vi "Start-Stop Remote Ping.vi"(8 "Error In":errorcluster, 10 "Start Remote Ping":bool, 11 "Test LNA in":refnum<class "TestLNA.lvclass">) -> (0 "Error Out":errorcluster, 3 "Test LNA out":refnum<class "TestLNA.lvclass">)   [LabVIEW 2014, in "TestLNA.lvlib" / "TestLNA.lvclass"]
doc: "Start or stop remote ping using iime delayed message."
uses:
  TestLNA.lvclass
  TestLNA.lvclass/TestLNA.ctl
  <vilib>/ActorFramework/Time-Delayed Send Message/Time-Delay Override Options.ctl
  Test LNA Messages/Remote Message Msg/Remote Message Msg.lvclass
  CSPP_Core/Actors/CS++BaseActor/CS++BaseActor.lvclass/CS++BaseActor.ctl
  <vilib>/ActorFramework/Actor/Actor.lvclass/Actor.ctl
  <vilib>/ActorFramework/Message Enqueuer/Message Enqueuer.lvclass/Message Enqueuer.ctl
  <vilib>/ActorFramework/Message Enqueuer/Init from Existing Queue.vi
  <vilib>/ActorFramework/Message Enqueuer/Message Enqueuer.lvclass
  <vilib>/ActorFramework/Actor/Actor.lvclass
  CSPP_Core/Actors/CS++BaseActor/CS++BaseActor.lvclass
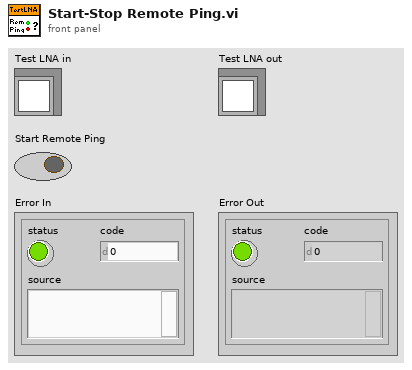
[diagram p1: front panel]
types:
  T1 = typedef "Time-Delay Override Options.ctl" = enum16{"Send next copy now", "Skip next scheduled copy", "Send next copy now and stop all further copies", "Stop all further copies"}
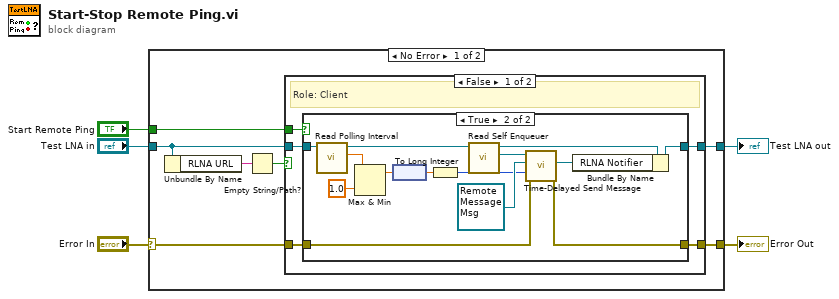
[diagram p0: block diagram]
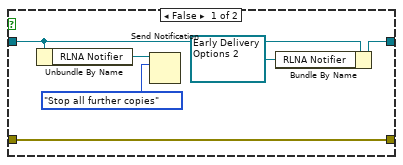
[diagram p2: hidden frame]
diagram:
  n1 = case shown="No Error" "Error In" {
    selector: "Error In" -> [w12 w40]
    tunnel: [w11 w40] -> w4
    tunnel: [w10 w39] -> w2
    tunnel: "Test LNA in" -> [w8 w39]
    tunnel: "Start Remote Ping" -> [w9 _]
    frame No Error {
      n2 = Unbundle By Name(w8) -> ("RLNA URL"=w7:string)
      n3 = Empty String/Path?(string/path=w7) -> (empty?=w6:bool)
      n4 = case shown="False" w6 {
        tunnel: w12 -> [w17 w37]
        tunnel: [w16 w37] -> w11
        tunnel: [w15 w38] -> w10
        tunnel: w9 -> [w14 _]
        tunnel: w8 -> [w13 w38]
        frame False {
          # "Role: Client"
          n5 = case shown="True" w14 {
            tunnel: w17 -> [w18 w34]
            tunnel: [w18 w33] -> w16
            tunnel: w13 -> [w22 w30]
            tunnel: [w21 w32] -> w15
            frame False {
              w20 = refnum<notifier> refnum items=["Send next copy now", "Skip next scheduled copy", "Send next copy now and stop all further copies", "Stop all further copies"] ("RAPing Notifier")
              n6 = Unbundle By Name(w22) -> ("RLNA Notifier"=w23:refnum<notifier>)
              n7 = Send Notification(notification=Time-Delay_Override_Options."Stop all further copies", notifier=w23) -> ()  [unwired: 1 in, 2 out]
              n8 = Bundle By Name(cluster=w22, "RLNA Notifier"=w20) -> (w21:refnum<class "TestLNA.lvclass">)
            }
            frame True {
              n9 = call "Read Polling Interval.vi"("CS++BaseActor in"=w30) -> ("Polling Interval"=w28:dbl[unit], "CS++BaseActor out"=w29:refnum<class "TestLNA.lvclass">)  [unwired: 8 in, 1 out]
              n10 = Max & Min(x=w28, y=dbl[unit] 1.0) -> (max(x,y)=w26:dbl[unit])  [unwired: 1 out]
              n11 = node(w26) -> (w25:dbl)
              n12 = To Long Integer(number=w25) -> (32bit integer=w24:i32)
              n13 = call <vilib>:"Read Self Enqueuer.vi"("Actor"=w29) -> ("Self Enqueuer"=w35:refnum<class "Message Enqueuer.lvclass">)  [unwired: 10 in]
              n14 = call <vilib>:"Time-Delayed Send Message.vi"("error in (no error)"=w34, "Milliseconds To Wait"=w24, "Message"=refnum<class "Remote Message Msg.lvclass"> refnum ("Ping Remote Actor Msg.lvclass"), "Message Enqueuer"=w35) -> ("error out"=w33:errorcluster, "Delivery Notifier"=w31:refnum<notifier>)  [unwired: 6 in]
              n15 = Bundle By Name(cluster=w29, "RLNA Notifier"=w31) -> (w32:refnum<class "TestLNA.lvclass">)
            }
          }
        }
        frame True {
          # "Role: Server"
        }
      }
    }
    frame Error {
    }
  }
  "Error Out" <- w4
  "Test LNA out" <- w2
